vi "CH_LM Utility Meter Information.vi"(0 "Meter Index":i32, 1 "Date Format (MDY)":T1, 2 "Time Stamp":timestamp format="%<%X\n%x>T", 5 "error in (no error)":errorcluster, 7 "Timeout / ms (3000)":i32=3000, 8 "Action (query)":bool, 9 "Lock Timeout / ms (1000)":i32=1000) -> (11 "Lock timed out":bool, 12 "Meter Type":T2, 13 "Serial Number":string, 14 "Meter Index":i32, 15 "Date Format":T1, 16 "Time Stamp":timestamp format="%<%X\n%x>T", 17 "Calibration Date":string, 19 "error out":errorcluster)   [LabVIEW 2012, in "CH_LM.lvlib"]
doc: "The command will set/query date and time maintained within the meter as well as the panel display date format used by the meter. Further more the calibration date, serial number and meter type (TOP or TO) is queried."
uses:
  CH_LM.lvlib
  CH_LM Meter Type.ctl
  CH_LM Date Format.ctl
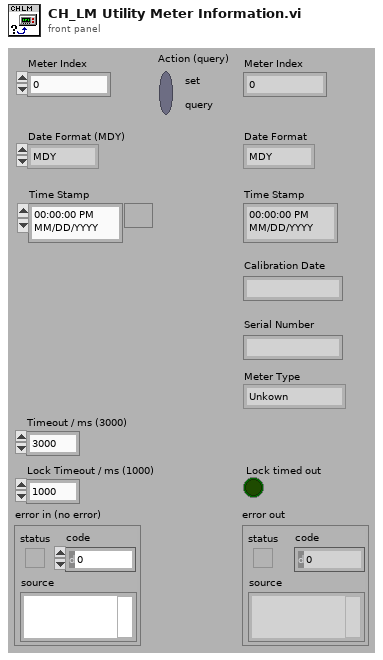
[diagram p1: front panel]
types:
  T1 = typedef "CH_LM.lvlib/CH_LM Date Format.ctl" = enum16{"MDY", "DMY"}
  T2 = typedef "CH_LM.lvlib/CH_LM Meter Type.ctl" = enum16{"Unkown", "TOP", "TO"}
  T3 = cluster{"second":i32, "minute":i32, "hour":i32, "day of month":i32, "month":i32, "year":i32, "day of week":i32, "day of year":i32, "is DST":i32}
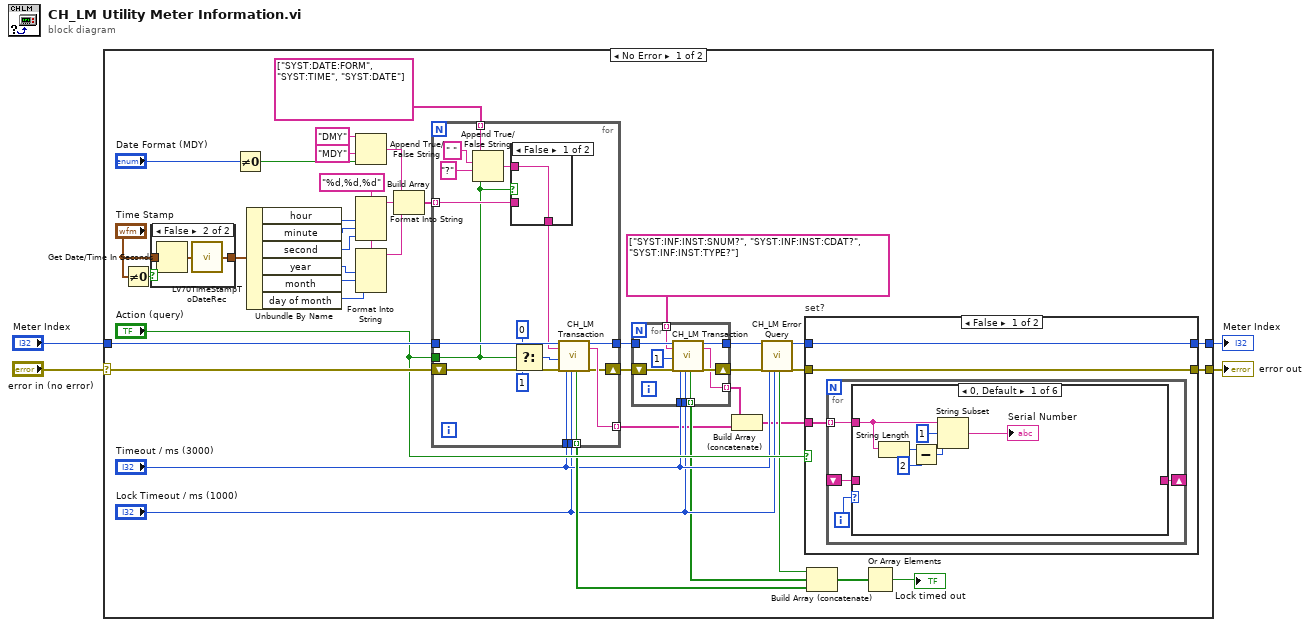
[diagram p0: block diagram]
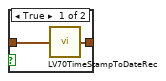
[diagram p2: hidden frame]
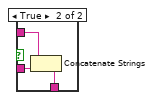
[diagram p3: hidden frame]
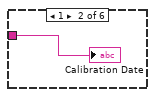
[diagram p4: hidden frame]
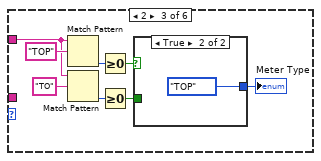
[diagram p5: hidden frame]
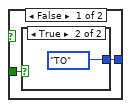
[diagram p6: hidden frame]
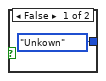
[diagram p7: hidden frame]
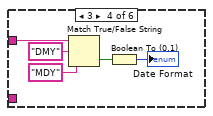
[diagram p8: hidden frame]
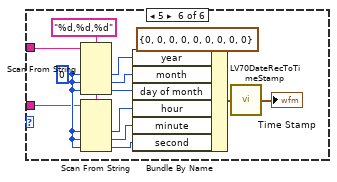
[diagram p10: hidden frame]
diagram:
  n1 = case shown="No Error" "error in (no error)" {
    selector: "error in (no error)" -> [w45 w131]
    tunnel: [w43 w131] -> w4
    tunnel: "Meter Index" -> [w44 w130]
    tunnel: [w42 w130] -> w1
    frame No Error {
      w29 = "%d,%d,%d" ("format string")
      n2 = Not Equal To 0?(x="Time Stamp") -> (x != 0?=w7:bool)
      n3 = case shown="False" w7 {
        tunnel: "Time Stamp" -> [w47 _]
        tunnel: [w46 w49] -> w5
        frame True {
          n4 = call <vilib>:"LV70TimeStampToDateRec.vi"("time stamp"=w47) -> ("date time rec"=w46:T3)
        }
        frame False {
          n5 = Get Date/Time In Seconds() -> (seconds since 1Jan1904=w48:timestamp)
          n6 = call <vilib>:"LV70TimeStampToDateRec.vi"("time stamp"=w48) -> ("date time rec"=w49:T3)
        }
      }
      n7 = Not Equal To 0?(x="Date Format (MDY)") -> (x != 0?=w27:bool)
      n8 = Unbundle By Name(w5) -> ("hour"=w35:i32, "minute"=w34:i32, "second"=w33:i32, "year"=w32:i32, "month"=w31:i32, "day of month"=w30:i32)
      n9 = Append True/False String(1:w27, 2:"MDY" ("false string"), 3:"DMY" ("true string")) -> (0:w22:string)  [unwired: 1 out]
      n10 = Format Into String(format string=w29, w35, w34, w33) -> (resulting string=w21:string)  [unwired: 2 in, 1 out]
      n11 = Format Into String(format string=w29, w32, w31, w30) -> (resulting string=w20:string)  [unwired: 2 in, 1 out]
      n12 = Build Array(w22, w21, w20) -> (w19:string[])
      n13 = for {
        tunnel: w44 -> [w76]
        tunnel: "Timeout / ms (3000)" -> [w75]
        tunnel: "Lock Timeout / ms (1000)" -> [w74]
        tunnel: "Action (query)" -> [w60]
        tunnel: [w73] -> w10 mode=indexing
        tunnel: [w68] -> w15
        tunnel: [w66] -> w37 mode=indexing
        tunnel: string[] ["SYST:DATE:FORM", "SYST:TIME", "SYST:DATE"] -> [w64] mode=indexing
        shift-right: [w67] -> w18
        shift-left: w45 -> [w77]
        tunnel: w19 -> [w63] mode=indexing
        n14 = Append True/False String(1:w60, 2:"?" ("true string"), 3:" ", 4:w64) -> (0:w62:string)
        n15 = case shown="False" w60 {
          tunnel: w63 -> [_ w81]
          tunnel: w62 -> [w78 w80]
          tunnel: [w78 w79] -> w61
          frame False {
          }
          frame True {
            n16 = Concatenate Strings(w80, w81) -> (w79:string)
          }
        }
        n17 = Select(t=0, s=w60, f=1 ("NofStrings (-1:all)")) -> (s? t:f=w70:i32)
        n18 = call "CH_LM Transaction.vi"("Meter Index"=w76, "Command String"=w61, "NofStrings (-1:all)"=w70, "error in (no error)"=w77, "Timeout / ms (3000)"=w75, "Lock Timeout / ms (1000)"=w74) -> ("Lock timed out"=w66:bool, "Meter Index"=w68:i32, "Response"=w73:string, "error out"=w67:errorcluster)  [unwired: 10 out]
      }
      n19 = for {
        tunnel: [w57] -> w16
        tunnel: w15 -> [w56]
        tunnel: "Timeout / ms (3000)" -> [w55]
        tunnel: "Lock Timeout / ms (1000)" -> [w54]
        tunnel: string[] ["SYST:INF:INST:SNUM?", "SYST:INF:INST:CDAT?", "SYST:INF:INST:TYPE?"] -> [w53] mode=indexing
        tunnel: [w51] -> w11 mode=indexing
        shift-right: [w58] -> w17
        shift-left: w18 -> [w59]
        tunnel: [w50] -> w9 mode=indexing
        n20 = call "CH_LM Transaction.vi"("Meter Index"=w56, "Command String"=w53, "NofStrings (-1:all)"=1, "error in (no error)"=w59, "Timeout / ms (3000)"=w55, "Lock Timeout / ms (1000)"=w54) -> ("Lock timed out"=w51:bool, "Meter Index"=w57:i32, "Response"=w50:string, "error out"=w58:errorcluster)  [unwired: 10 out]
      }
      n21 = Build Array (concatenate)(w9, w10) -> (w8:string[])
      n22 = call "CH_LM Error Query.vi"("Meter Index"=w16, "error in (no error)"=w17, "Timeout / ms (3000)"="Timeout / ms (3000)", "Lock Timeout / ms (1000)"="Lock Timeout / ms (1000)") -> ("Lock timed out"=w38:bool, "Meter Index"=w40:i32, "error out"=w39:errorcluster)  [unwired: 13 out]
      n23 = case "set?" shown="False" "Action (query)" {
        tunnel: w39 -> [w83 w129]
        tunnel: [w83 w129] -> w43
        tunnel: w40 -> [w84 w128]
        tunnel: [w84 w128] -> w42
        tunnel: w8 -> [w82 _]
        frame False {
          n24 = for {
            tunnel: w82 -> [w87] mode=indexing
            shift-right: [w86] -> _
            shift-left: _ -> [w85]
            i -> [w88]
            n25 = case shown="0, Default" w88 {
              tunnel: w87 -> [w92 w95 w99 w113 w114 w127]
              tunnel: [_ _ _ _ w114 _] -> w86
              tunnel: w85 -> [_ _ _ _ _ w125]
              frame 0, Default {
                n26 = String Length(string=w92) -> (length=w91:i32)
                n27 = Subtract(x=w91, y=2) -> (x-y=w89:i32)
                n28 = String Subset(string=w92, offset (0)=1, length (rest)=w89) -> (substring=→"Serial Number":string)
              }
              frame 1 {
                "Calibration Date" <- w95
              }
              frame 2 {
                n29 = Match Pattern(string=w99, regular expression="TOP") -> (offset past match=w101:i32)  [unwired: 4 out]
                n30 = Match Pattern(string=w99, regular expression="TO") -> (offset past match=w102:i32)  [unwired: 4 out]
                n31 = Greater Or Equal To 0?(x=w101) -> (x >= 0?=w98:bool)
                n32 = Greater Or Equal To 0?(x=w102) -> (x >= 0?=w97:bool)
                n33 = case shown="True" w98 {
                  tunnel: w97 -> [w105 _]
                  tunnel: [w104 CH_LM_Meter_Type."TOP" ("Meter Type")] -> w96
                  frame False {
                    n34 = case shown="True" w105 {
                      tunnel: [CH_LM_Meter_Type."Unkown" ("Meter Type") CH_LM_Meter_Type."TO" ("Meter Type")] -> w104
                      frame False {
                      }
                      frame True {
                      }
                    }
                  }
                  frame True {
                  }
                }
                "Meter Type" <- w96
              }
              frame 3 {
                n35 = Match True/False String(2:"MDY" ("false string"), 3:"DMY" ("true string"), 4:w113) -> (0:w112:bool)  [unwired: 1 out]
                n36 = Boolean To (0,1)(Boolean=w112) -> (0, 1=→"Date Format":i16)
              }
              frame 4 {
              }
              frame 5 {
                w124 = "%d,%d,%d" ("format string")
                w126 = 0 ("default value 1")
                n37 = Scan From String(format string=w124, input string=w127, default 1=w126, default 2=w126, default 3=w126) -> (output 1=w123:i32, output 2=w122:i32, output 3=w121:i32)  [unwired: 2 in, 3 out]
                n38 = Scan From String(format string=w124, input string=w125, default 1=w126, default 2=w126, default 3=w126) -> (output 1=w120:i32, output 2=w119:i32, output 3=w118:i32)  [unwired: 2 in, 3 out]
                n39 = Bundle By Name(cluster=T3 {"second"=0, "minute"=0, "hour"=0, "day of month"=0, "month"=0, "year"=0, "day of week"=0, "day of year"=0, "is DST"=0} ("date time rec"), "year"=w123, "month"=w122, "day of month"=w121, "hour"=w120, "minute"=w119, "second"=w118) -> (w115:T3)
                n40 = call <vilib>:"LV70DateRecToTimeStamp.vi"("date time rec"=w115) -> ("Time Stamp"=→"Time Stamp":timestamp)
              }
            }
          }
        }
        frame True {
        }
      }
      n41 = Build Array (concatenate)(w38, w11, w37) -> (w36:bool[])
      n42 = Or Array Elements(Boolean array=w36) -> (logical OR=→"Lock timed out":bool)
    }
    frame Error {
    }
  }
  "error out" <- w4
  "Meter Index" <- w1
